vi "Init Divider.vi"(4 "Maximal size":i16[](array[numeric]), 5 "Label":string, 6 "Minimal size":i16[](array[numeric]), 7 "Vertical? [F, hor.]":bool, 8 "error in (no error)":errorcluster, 9 "Relative size":dbl[](array[numeric]), 10 "Items":refnum<class "IObject.lvclass">[](array[class]), 11 "Divider in":refnum<class "Divider.lvclass">) -> (0 "error out":errorcluster, 3 "Divider out":refnum<class "Divider.lvclass">)   [LabVIEW 2013, in "Divider.lvclass"]
doc: "Copyright 2018, Wiebe Walstra, wiebe@carya.nl."
uses:
  Divider.lvclass
  IObject.lvclass
  Divider.lvclass/Divider.ctl
  IContainer.lvclass
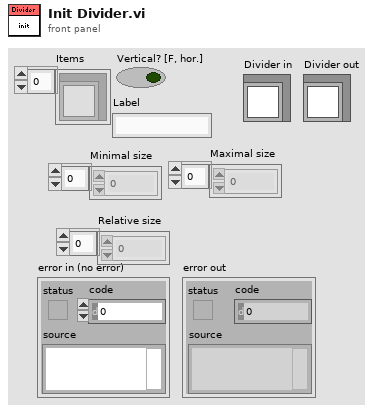
[diagram p1: front panel]
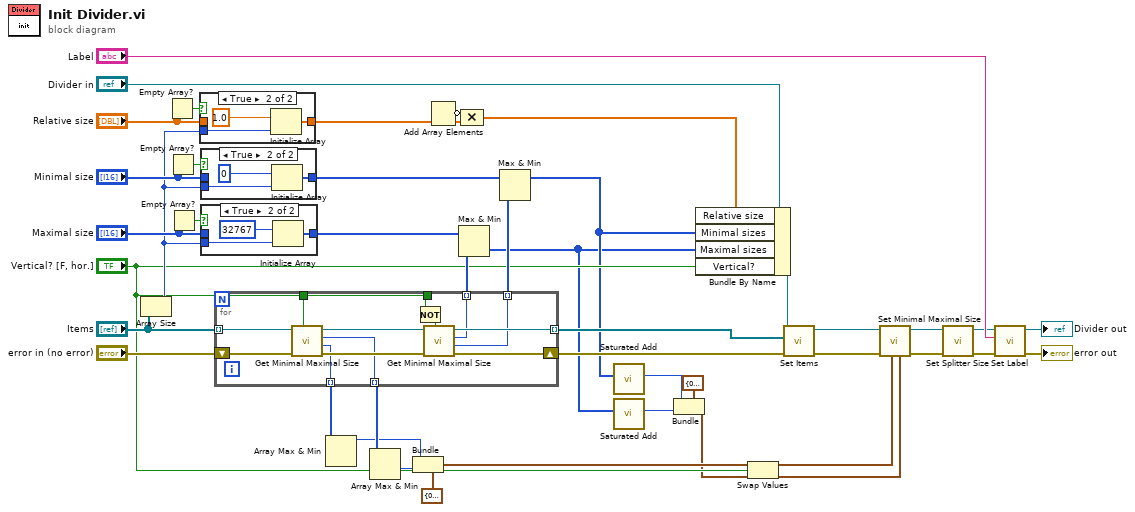
[diagram p0: block diagram]
diagram:
  n1 = Array Size(array="Items") -> (size(s)=w33:i32)
  n2 = Empty Array?(array="Relative size") -> (empty?=w40:bool)
  n3 = Empty Array?(array="Minimal size") -> (empty?=w38:bool)
  n4 = Empty Array?(array="Maximal size") -> (empty?=w35:bool)
  n5 = case shown="True" w40 {
    tunnel: w33 -> [_ w48]
    tunnel: [w45 w46] -> w37
    tunnel: "Relative size" -> [w45 _]
    frame False {
    }
    frame True {
      n6 = Initialize Array(1.0 ("element"), w48) -> (w46:dbl[])
    }
  }
  n7 = case shown="True" w38 {
    tunnel: w33 -> [_ w52]
    tunnel: [w49 w50] -> w19
    tunnel: "Minimal size" -> [w49 _]
    frame False {
    }
    frame True {
      n8 = Initialize Array(i16 0 ("element"), w52) -> (w50:i16[])
    }
  }
  n9 = case shown="True" w35 {
    tunnel: w33 -> [_ w56]
    tunnel: [w53 w54] -> w18
    tunnel: "Maximal size" -> [w53 _]
    frame False {
    }
    frame True {
      n10 = Initialize Array(i16 32767 ("element"), w56) -> (w54:i16[])
    }
  }
  n11 = for {
    tunnel: "Items" -> [w63] mode=indexing
    tunnel: [w69] -> w27 mode=indexing
    shift-right: [w68] -> w25
    shift-left: "error in (no error)" -> [w60]
    tunnel: [w67] -> w24 mode=indexing
    tunnel: [w66] -> w23 mode=indexing
    tunnel: "Vertical? [F, hor.]" -> [w65]
    tunnel: "Vertical? [F, hor.]" -> [w59]
    tunnel: [w58] -> w15 mode=indexing
    tunnel: [w57] -> w13 mode=indexing
    n12 = call-dynamic "Get Minimal Maximal Size.vi"("Vertical? [F, hor.]"=w59, "error in (no error)"=w60, "IObject in"=w63) -> ("error out"=w61:errorcluster, "Minimal size"=w57:i16, "Maximal size"=w58:i16, "IObject out"=w62:refnum<class "IObject.lvclass">)  [unwired: 5 in]
    n13 = Not(x=w65) -> (.not. x?=w64:bool)
    n14 = call-dynamic "Get Minimal Maximal Size.vi"("Vertical? [F, hor.]"=w64, "error in (no error)"=w61, "IObject in"=w62) -> ("error out"=w68:errorcluster, "Minimal size"=w66:i16, "Maximal size"=w67:i16, "IObject out"=w69:refnum<class "IObject.lvclass">)  [unwired: 5 in]
  }
  n15 = Array Max & Min(array=w13) -> (max value=w12:i16)  [unwired: 3 out]
  n16 = Array Max & Min(array=w15) -> (min value=w11:i16)  [unwired: 3 out]
  n17 = Bundle(cluster=cluster{"Minimal":i16, "Maximal":i16} {"Minimal"=0, "Maximal"=32767} ("Vertical"), "Minimal"=w12, "Maximal"=w11) -> (w2:cluster{"Minimal":i16, "Maximal":i16})
  n18 = Add Array Elements(numeric array=w37) -> (sum=w42:dbl)
  n19 = Max & Min(x=w18, y=w24) -> (min(x,y)=w6:i16[])  [unwired: 1 out]
  n20 = Compound Arithmetic op=MULTIPLY(invert w42, w37) -> (w16:dbl[])
  n21 = Max & Min(x=w19, y=w23) -> (max(x,y)=w7:i16[])  [unwired: 1 out]
  n22 = call "Saturated Add.vi"("Sizes"=w7) -> ("Sum"=w4:i16)  [unwired: 10 in]
  n23 = call "Saturated Add.vi"("Sizes"=w6) -> ("Sum"=w3:i16)  [unwired: 10 in]
  n24 = Bundle(cluster=cluster{"Minimal":i16, "Maximal":i16} {"Minimal"=0, "Maximal"=32767} ("Vertical"), "Minimal"=w4, "Maximal"=w3) -> (w1:cluster{"Minimal":i16, "Maximal":i16})
  n25 = Bundle By Name(cluster="Divider in", "Relative size"=w16, "Minimal sizes"=w7, "Maximal sizes"=w6, "Vertical?"="Vertical? [F, hor.]") -> (w44:refnum<class "Divider.lvclass">)
  n26 = Swap Values(12:w2, 13:"Vertical? [F, hor.]", 14:w1) -> (1:w8:cluster{"Minimal":i16, "Maximal":i16}, 3:w9:cluster{"Minimal":i16, "Maximal":i16})
  n27 = call "Set Items.vi"("error in (no error)"=w25, "Items"=w27, "IContainer in"=w44) -> ("error out"=w43:errorcluster, "IContainer out"=w21:refnum<class "Divider.lvclass">)  [unwired: 7 in]
  n28 = call "Set Minimal Maximal Size.vi"("Vertical"=w9, "Horizontal"=w8, "error in (no error)"=w43, "MMI Scaling in"=w21) -> ("error out"=w22:errorcluster, "MMI Scaling out"=w20:refnum<class "Divider.lvclass">)  [unwired: 6 in]
  n29 = call "Set Splitter Size.vi"("error in (no error)"=w22, "Divider in"=w20) -> ("error out"=w29:errorcluster, "Divider out"=w28:refnum<class "Divider.lvclass">)  [unwired: 8 in]
  n30 = call "Set Label.vi"("error in (no error)"=w29, "Label"="Label", "MMI Scaling in"=w28) -> ("error out"=→"error out":errorcluster, "MMI Scaling out"=→"Divider out":refnum<class "Divider.lvclass">)  [unwired: 7 in]
